vi "Calculate Close Tab Button Position.vi"(8 "error in":errorcluster, 10 "Tab Control Reference In":refnum<vi>, 11 "Close Tab Button Reference In":refnum<vi>) -> (0 "error out":errorcluster, 1 "Button Position":i32, 2 "Tab Control Reference Out":refnum<vi>, 3 "Close Tab Button Reference Out":refnum<vi>)   [LabVIEW 2017, in "DTacq Plot Display Library.lvlib"]
uses:
  DTacq Plot Display Library.lvlib
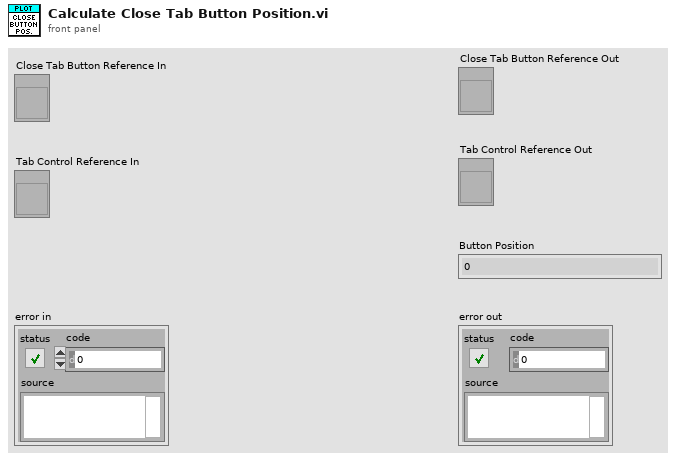
[diagram p1: front panel]
types:
  T1 = enum32{"Page 1", "Page 2", "Page 3", "Page 4", "Page 5", "Page 6"}
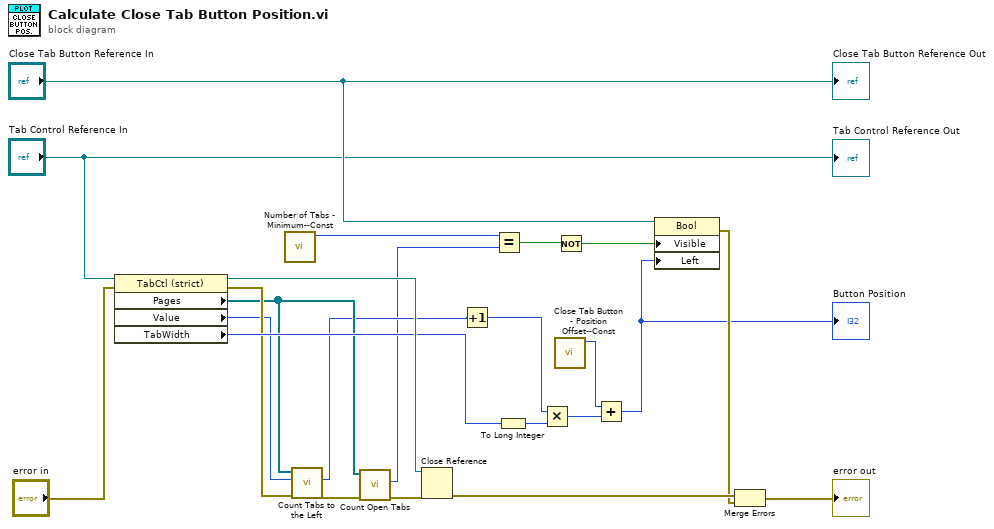
[diagram p0: block diagram]
diagram:
  n1 = property class="TabCtl (strict)"(reference="Tab Control Reference In", error in="error in") -> (reference out=w20:refnum<vi>, error out=w7:errorcluster, "Pages"=w5:refnum<vi>[], "Value"=w6:T1, "TabWidth"=w15:u32)
  n2 = call "Number of Tabs - Minimum--Const.vi"() -> ("Minimum Tabs"=w10:i32)  [unwired: 11 in]
  n3 = call "Count Tabs to the Left.vi"("error in"=w7, "Current Tab"=w6, "Tab Pages References In"=w5) -> ("error out"=w4:errorcluster, "Number of Tabs to the Left"=w2:i32)  [unwired: 6 in, 1 out]
  n4 = call "Count Open Tabs.vi"("error in"=w4, "Tab Pages References In"=w5) -> ("error out"=w3:errorcluster, "Number of Open Tabs"=w1:i32)  [unwired: 7 in, 1 out]
  n5 = Close Reference(reference=w20, error in (no error)=w3) -> (error out=w18:errorcluster)
  n6 = Increment(x=w2) -> (x+1=w13:i32)
  n7 = Equal?(x=w10, y=w1) -> (x = y?=w9:bool)
  n8 = To Long Integer(number=w15) -> (32bit integer=w14:i32)
  n9 = Multiply(x=w13, y=w14) -> (x*y=w23:i32)
  n10 = call "Close Tab Button - Position Offset--Const.vi"() -> ("Position Offset"=w22:i32)  [unwired: 11 in]
  n11 = Not(x=w9) -> (.not. x?=w8:bool)
  n12 = Add(x=w22, y=w23) -> (x+y=w11:i32)
  "Button Position" <- w11
  n13 = property class="Bool"(reference="Close Tab Button Reference In", "Visible"=w8, "Left"=w11) -> (error out=w17:errorcluster)  [unwired: 1 in, 1 out]
  n14 = Merge Errors(w18, w17) -> (→"error out":errorcluster)
  "Close Tab Button Reference Out" <- "Close Tab Button Reference In"
  "Tab Control Reference Out" <- "Tab Control Reference In"
